vi "UART Configure.vi"(8 "Error In":errorcluster, 9 "UART Settings":T1={"Baud (ticks)"=1736, "CharacterSize"=8, "Parity"=enum."None", "Stop Bits"=enum."1.0", "Spacing (ticks)"=0}, 10 "UART Host Buffer Size":u32=1000, 11 "FPGA Interface":refnum<k20>) -> (0 "Error Out":errorcluster, 3 "FPGA Interface Out":refnum<k20>)   [LabVIEW 2015]
uses:
  <vilib>/rvi/interface/common/niFpgaWaitOnOcc.vi
  <vilib>/Utility/error.llb/Error Cluster From Error Code.vi
  <vilib>/rvi/errors/niLvFpgaAdjustHostInterfaceError.vi
  <vilib>/rvi/interface/nirviMethod/nirviMethod.xnode
  <vilib>/rvi/interface/nirviReadWriteControl/nirviReadWriteControl.xnode
  <vilib>/FPGAPlugInAG/Dynamic/niLvFpga_ConfigureFifo_Dynamic.vi
  <vilib>/rvi/errors/niLvFpgaMergeErrorWithErrorCode.vi
  NiFpgaLv.dll
  <vilib>/rvi/interface/Simulation/niFpgaSimulationCallBeginRW.vi
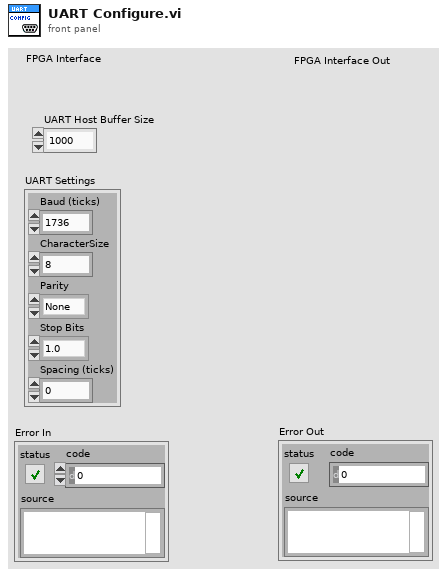
[diagram p1: front panel]
types:
  T1 = cluster{"Baud (ticks)":u32, "CharacterSize":u8, "Parity":enum8{"None", "Even", "Odd"}, "Stop Bits":enum8{"1.0", "1.5", "2.0"}, "Spacing (ticks)":u32}
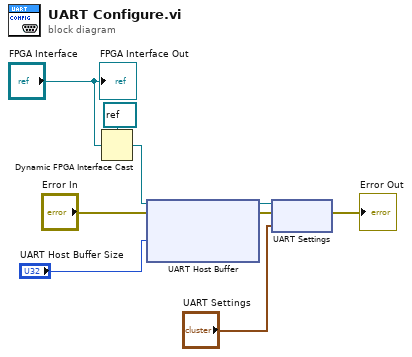
[diagram p0: block diagram]
diagram:
  n1 = Dynamic FPGA Interface Cast(Session In=refnum<k20> refnum ("FPGA Interface"), Type="FPGA Interface") -> (Session Out=w1:refnum<k20>)
  n2 = xnode "UART Host Buffer"("FPGA VI Reference In"=w1, "error in"="Error In", "Requested Depth"="UART Host Buffer Size") -> ("FPGA VI Reference Out"=w9:refnum<k20>, "error out"=w8:errorcluster)  [unwired: 1 out]
  n3 = xnode "UART Settings"("FPGA VI Reference In"=w9, "error in"=w8, "Settings"="UART Settings") -> ("error out"=→"Error Out":errorcluster)  [unwired: 1 out]
  "FPGA Interface Out" <- "FPGA Interface"
